vi "Grid NextPositionCol.vi"(6 "表サイズ(縦x横)":i32[](array[numeric]), 7 "VKey(Right)":T1=enum."Right" caption="VKey", 8 "error in (no error)":errorcluster caption="エラー入力（エラーなし）", 10 "EditPos入力":T2 caption="EditPos", 11 "ref.表":refnum<vi>) -> (0 "error out":errorcluster caption="エラー出力", 2 "EditPos出力":T2 caption="EditPos", 3 "ref.表(copy)":refnum<vi>)   [LabVIEW 2014]
uses:
  <vilib>/Utility/miscctls.llb/LVRowAndColumnTypeDef.ctl
  <vilib>/event_ctls.llb/eventvkey.ctl
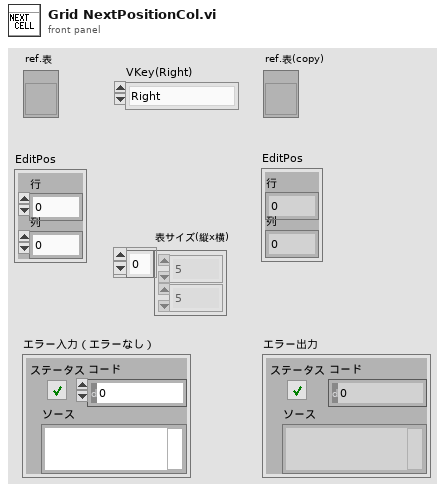
[diagram p1: front panel]
types:
  T1 = typedef "eventvkey.ctl" = enum16{"ASCII", "Enter", "Return", "Shift", "Ctrl", "Alt", "Cmd", "Opt", "Caps", "NumLock", "Clear", "Break", "Up", "Down", "Left", "Right", "Insert", "Delete", "Home", "End", "PageUp", "PageDown", "Escape", "Help", "Pause", "ScrollLock", "F1", "F2", "F3", "F4", "F5", "F6", "F7", "F8", "F9", "F10", "F11", "F12", "F13", "F14", "F15", "F16", "F17", "F18", "F19", "F20", "F21", "F22", "F23", "F24", "Play", "VolumeUp", "VolumeDown", "Mute", "Two Byte Char"}
  T2 = typedef "LVRowAndColumnTypeDef.ctl" = cluster{"Row":i32, "Column":i32}
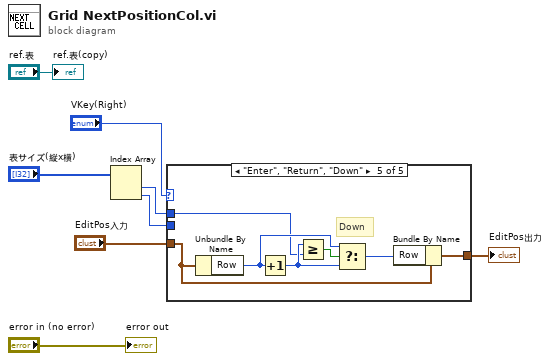
[diagram p0: block diagram]
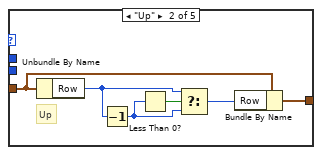
[diagram p3: hidden frame]
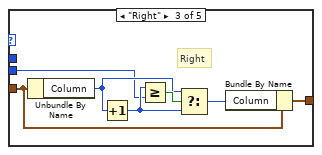
[diagram p4: hidden frame]
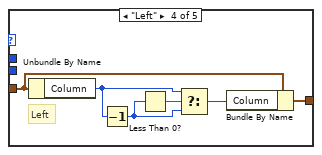
[diagram p5: hidden frame]
diagram:
  n1 = Index Array(array="表サイズ(縦x横)") -> (element #1=w5:i32, element #2=w4:i32)  [unwired: 2 in]
  n2 = case shown="\"Enter\", \"Return\", \"Down\"" "VKey(Right)" {
    tunnel: [w9 w14 w22 w23 w30] -> w8
    tunnel: "EditPos入力" -> [w9 w15 w21 w25 w32]
    tunnel: w5 -> [_ _ _ _ w29]
    tunnel: w4 -> [_ _ w16 _ _]
    frame Default {
    }
    frame "Up" {
      # "Up"
      n3 = Unbundle By Name(w15) -> ("Row"=w10:i32)
      n4 = Decrement(x=w10) -> (x-1=w12:i32)
      n5 = Less Than 0?(x=w12) -> (x < 0?=w13:bool)
      n6 = Select(t=w10, s=w13, f=w12) -> (s? t:f=w11:i32)
      n7 = Bundle By Name(cluster=w15, "Row"=w11) -> (w14:T2)
    }
    frame "Right" {
      # "Right"
      n8 = Unbundle By Name(w21) -> ("Column"=w19:i32)
      n9 = Increment(x=w19) -> (x+1=w18:i32)
      n10 = Greater Or Equal?(x=w18, y=w16) -> (x >= y?=w20:bool)
      n11 = Select(t=w19, s=w20, f=w18) -> (s? t:f=w17:i32)
      n12 = Bundle By Name(cluster=w21, "Column"=w17) -> (w22:T2)
    }
    frame "Left" {
      # "Left"
      n13 = Unbundle By Name(w25) -> ("Column"=w27:i32)
      n14 = Decrement(x=w27) -> (x-1=w26:i32)
      n15 = Less Than 0?(x=w26) -> (x < 0?=w28:bool)
      n16 = Select(t=w27, s=w28, f=w26) -> (s? t:f=w24:i32)
      n17 = Bundle By Name(cluster=w25, "Column"=w24) -> (w23:T2)
    }
    frame "Enter", "Return", "Down" {
      # "Down"
      n18 = Unbundle By Name(w32) -> ("Row"=w34:i32)
      n19 = Increment(x=w34) -> (x+1=w33:i32)
      n20 = Greater Or Equal?(x=w33, y=w29) -> (x >= y?=w35:bool)
      n21 = Select(t=w34, s=w35, f=w33) -> (s? t:f=w31:i32)
      n22 = Bundle By Name(cluster=w32, "Row"=w31) -> (w30:T2)
    }
  }
  "EditPos出力" <- w8
  "ref.表(copy)" <- "ref.表"
  "error out" <- "error in (no error)"
